vi "CreateBricks.vi"(8 "error in":errorcluster, 11 "class data in":refnum<class "Game.lvclass">) -> (0 "error out":errorcluster, 3 "class data out":refnum<class "Game.lvclass">)   [LabVIEW 2010, in "Labricks.lvlib" / "Game.lvclass"]
uses:
  Game.lvclass
  Game.lvclass/Game.ctl
  Brick_class/Brick.lvclass
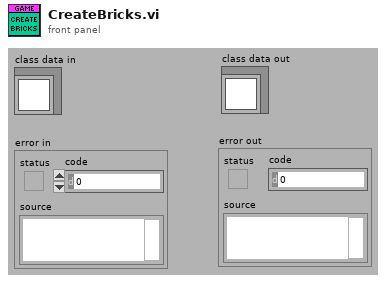
[diagram p1: front panel]
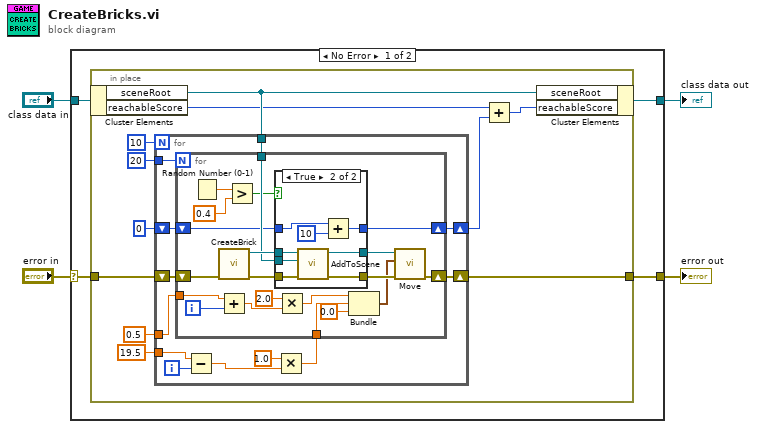
[diagram p0: block diagram]
diagram:
  n1 = case shown="No Error" "error in" {
    selector: "error in" -> [w7 w64]
    tunnel: [w8 w64] -> w4
    tunnel: "class data in" -> [w6 w63]
    tunnel: [w5 w63] -> w2
    frame No Error {
      n2 = in-place {
        in-place-border: [w17] -> w8
        in-place-border: w7 -> [w13]
        n3 = in-place-cluster #1(w6) -> ("sceneRoot"=w11:refnum<class "SceneRoot.lvclass">, "reachableScore"=w10:i32)
        n4 = for {
          N: 10 -> [_]
          tunnel: w11 -> [w31]
          tunnel: 20 -> [w30]
          tunnel: 19.5 -> [w27]
          shift-right: [w25] -> w17
          shift-left: w13 -> [w24]
          tunnel: 0.5 -> [w23]
          shift-right: [w21] -> w12
          shift-left: 0 -> [w22]
          i -> [w20]
          n5 = Subtract(x=w27, y=w20) -> (x-y=w28:dbl)
          n6 = Multiply(x=1.0, y=w28) -> (x*y=w26:dbl)
          n7 = for {
            N: w30 -> [_]
            tunnel: w31 -> [w49]
            tunnel: w26 -> [w44]
            shift-right: [w41] -> w25
            shift-left: w24 -> [w40]
            tunnel: w23 -> [w38]
            shift-right: [w36] -> w21
            shift-left: w22 -> [w37]
            i -> [w32]
            n8 = Random Number (0-1)() -> (number: 0 to 1=w34:dbl)
            n9 = call "CreateBrick.vi"("error in (no error)"=w40) -> ("error out"=w51:errorcluster, "class data out"=w50:refnum<class "Brick.lvclass">)  [unwired: 9 in]
            n10 = Add(x=w38, y=w32) -> (x+y=w39:dbl)
            n11 = Greater?(x=w34, y=0.4) -> (0:w35:bool)
            n12 = case shown="True" w35 {
              tunnel: w51 -> [w52 w62]
              tunnel: w50 -> [w53 w61]
              tunnel: w49 -> [_ w60]
              tunnel: [w53 w59] -> w48
              tunnel: [w52 w58] -> w47
              tunnel: w37 -> [w54 w57]
              tunnel: [w54 w56] -> w36
              frame False {
              }
              frame True {
                n13 = call-dynamic "AddToScene.vi"("error in (no error)"=w62, "sceneRoot in"=w60, "class data in"=w61) -> ("error out"=w58:errorcluster, "class data out"=w59:refnum<class "Brick.lvclass">)  [unwired: 7 in]
                n14 = Add(x=w57, y=10 ("x")) -> (x+y=w56:i32)
              }
            }
            n15 = Multiply(x=2.0, y=w39) -> (x*y=w43:dbl)
            n16 = Bundle(w43, w44, 0.0) -> (w46:cluster{dbl, dbl, dbl})  [unwired: 1 in]
            n17 = call-dynamic "Move.vi"("error in (no error)"=w47, "targetCoords in"=w46, "class data in"=w48) -> ("error out"=w41:errorcluster)  [unwired: 7 in, 1 out]
          }
        }
        n18 = Add(x=w10, y=w12) -> (x+y=w9:i32)
        n19 = in-place-cluster #1("sceneRoot"=w11, "reachableScore"=w9) -> (w5:refnum<class "Game.lvclass">)
      }
    }
    frame Error {
    }
  }
  "class data out" <- w2
  "error out" <- w4
